vi "getTestTimingInfo.vi"(8 "error in":errorcluster, 11 "TestRunner in":refnum<class "TestRunner.lvclass">) -> (0 "error out":errorcluster, 1 "Start Time":timestamp, 2 "Stop Time":timestamp, 3 "TestRunner out":refnum<class "TestRunner.lvclass">)   [LabVIEW 2013, in "TestRunner.lvclass"]
uses:
  TestRunner.lvclass
  TestRunner.lvclass/TestRunner.ctl
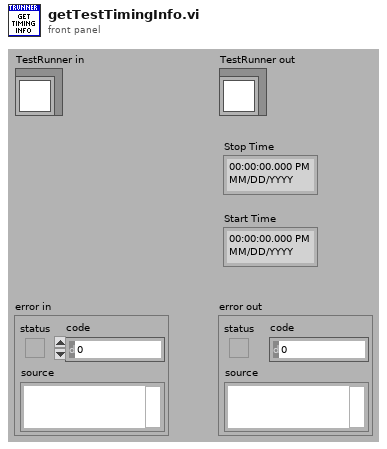
[diagram p1: front panel]
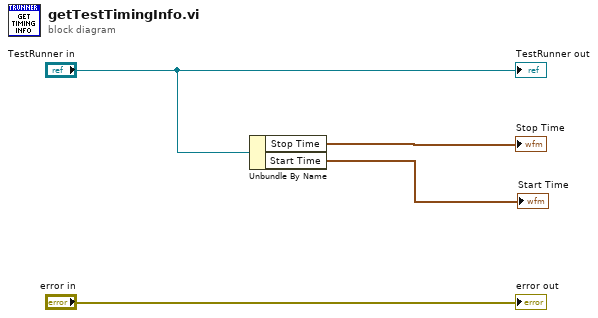
[diagram p0: block diagram]
diagram:
  n1 = Unbundle By Name("TestRunner in") -> ("Stop Time"=→"Stop Time":timestamp, "Start Time"=→"Start Time":timestamp)
  "TestRunner out" <- "TestRunner in"
  "error out" <- "error in"
